vi "sub vi - Syringe Settings.vi"(7 "VISA resource name":refnum<visa-resource-name>="COM11", 9 "Flow Rate (ul/min)":dbl=100.0, 10 "Force (1-100)":dbl=100.0, 11 "Diameter (mm)":dbl=100.0) -> (0 "Accumulated Volume (ul)":dbl format="%#_6f", 1 "Flow Rate (ul/min)":dbl format="%#_6f", 2 "force setting (0-100)":dbl format="%#_6f", 3 "Diameter (mm)":dbl format="%#_6f")   [LabVIEW 2010]
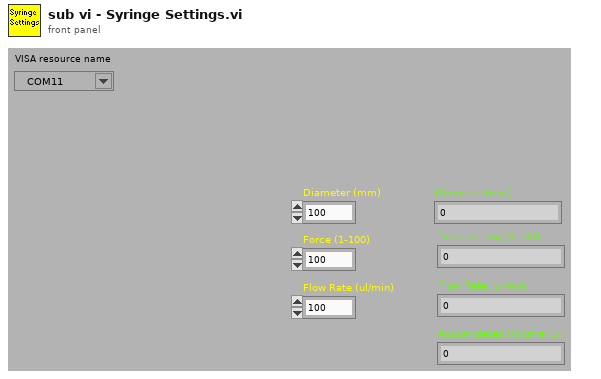
[diagram p1: front panel]
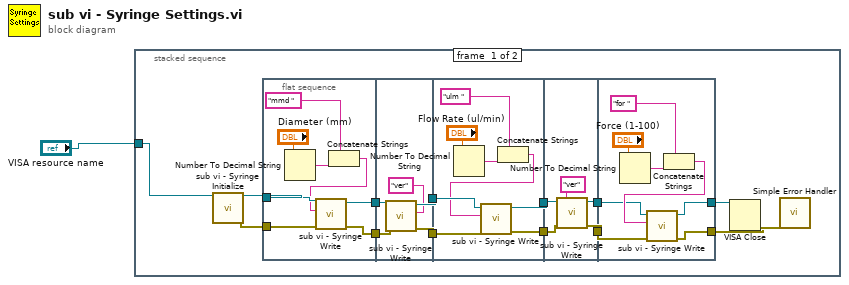
[diagram p0: block diagram]
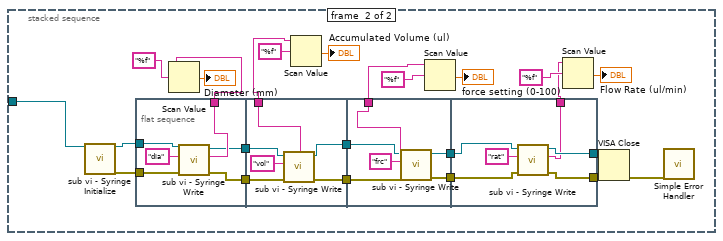
[diagram p2: hidden frame]
diagram:
  n1 = stacked-sequence {
    tunnel: "VISA resource name" -> [w2 w50]
    frame #0 {
      n2 = call "sub vi - Syringe Initialize.vi"("VISA resource name"=w2) -> ("VISA resource name out"=w6:refnum<visa-resource-name>, "error out"=w5:errorcluster)  [unwired: 13 out]
      n3 = flat-sequence {
        tunnel: w6 -> [w23]
        tunnel: w5 -> [w22]
        tunnel: [w21] -> w15
        tunnel: [w20] -> w14
        tunnel: w15 -> [w27]
        tunnel: w14 -> [w28]
        tunnel: [w26] -> w13
        tunnel: [w25] -> w12
        tunnel: w13 -> [w35]
        tunnel: w12 -> [w36]
        tunnel: [w30] -> w11
        tunnel: [w29] -> w10
        tunnel: w11 -> [w37]
        tunnel: w10 -> [w40]
        tunnel: [w38] -> w9
        tunnel: [w39] -> w8
        tunnel: [w42] -> w3
        tunnel: [w43] -> w4
        tunnel: w9 -> [w44]
        tunnel: w8 -> [w45]
        frame #0 {
          n4 = Number To Decimal String(number="Diameter (mm)") -> (decimal integer string=w17:string)  [unwired: 1 out]
          n5 = Concatenate Strings("mmd " ("string"), w17) -> (w16:string)
          n6 = call "sub vi - Syringe Write.vi"("error out"=w22, "Command"=w16, "VISA resource name out"=w23) -> ("error out 2"=w20:errorcluster, "VISA resource name out 2"=w21:refnum<visa-resource-name>)  [unwired: 7 out]
        }
        frame #1 {
          n7 = call "sub vi - Syringe Write.vi"("error out"=w28, "Command"="ver", "VISA resource name out"=w27) -> ("error out 2"=w25:errorcluster, "VISA resource name out 2"=w26:refnum<visa-resource-name>)  [unwired: 7 out]
        }
        frame #2 {
          n8 = Number To Decimal String(number="Flow Rate (ul/min)") -> (decimal integer string=w32:string)  [unwired: 1 out]
          n9 = Concatenate Strings("ulm " ("string"), w32) -> (w31:string)
          n10 = call "sub vi - Syringe Write.vi"("error out"=w36, "Command"=w31, "VISA resource name out"=w35) -> ("error out 2"=w29:errorcluster, "VISA resource name out 2"=w30:refnum<visa-resource-name>)  [unwired: 7 out]
        }
        frame #3 {
          n11 = call "sub vi - Syringe Write.vi"("error out"=w40, "Command"="ver", "VISA resource name out"=w37) -> ("error out 2"=w39:errorcluster, "VISA resource name out 2"=w38:refnum<visa-resource-name>)  [unwired: 7 out]
        }
        frame #4 {
          n12 = Number To Decimal String(number="Force (1-100)") -> (decimal integer string=w48:string)  [unwired: 1 out]
          n13 = Concatenate Strings("for " ("string"), w48) -> (w46:string)
          n14 = call "sub vi - Syringe Write.vi"("error out"=w45, "Command"=w46, "VISA resource name out"=w44) -> ("error out 2"=w42:errorcluster, "VISA resource name out 2"=w43:refnum<visa-resource-name>)  [unwired: 7 out]
        }
      }
      n15 = VISA Close(VISA resource name=w4, error in (no error)=w3) -> (error out=w7:errorcluster)
      n16 = call <vilib>:"Simple Error Handler.vi"("error in (no error)"=w7) -> ()  [unwired: 1 in, 8 out]
    }
    frame #1 {
      n17 = call "sub vi - Syringe Initialize.vi"("VISA resource name"=w50) -> ("VISA resource name out"=w55:refnum<visa-resource-name>, "error out"=w54:errorcluster)  [unwired: 13 out]
      n18 = flat-sequence {
        tunnel: [w78] -> w62
        tunnel: w55 -> [w77]
        tunnel: w54 -> [w76]
        tunnel: [w75] -> w73
        tunnel: [w74] -> w72
        tunnel: [w84] -> w57
        tunnel: w73 -> [w83]
        tunnel: w72 -> [w82]
        tunnel: [w81] -> w71
        tunnel: [w80] -> w70
        tunnel: [w88] -> w56
        tunnel: w71 -> [w87]
        tunnel: w70 -> [w86]
        tunnel: [w90] -> w69
        tunnel: [w89] -> w68
        tunnel: [w95] -> w63
        tunnel: [w96] -> w64
        tunnel: w69 -> [w93]
        tunnel: w68 -> [w94]
        tunnel: [w92] -> w51
        frame #0 {
          n19 = call "sub vi - Syringe Write.vi"("error out"=w76, "Command"="dia", "VISA resource name out"=w77) -> ("error out 2"=w74:errorcluster, "Return String"=w78:string, "VISA resource name out 2"=w75:refnum<visa-resource-name>)  [unwired: 6 out]
        }
        frame #1 {
          n20 = call "sub vi - Syringe Write.vi"("error out"=w82, "Command"="vol", "VISA resource name out"=w83) -> ("error out 2"=w81:errorcluster, "Return String"=w84:string, "VISA resource name out 2"=w80:refnum<visa-resource-name>)  [unwired: 6 out]
        }
        frame #2 {
          n21 = call "sub vi - Syringe Write.vi"("error out"=w87, "Command"="frc", "VISA resource name out"=w86) -> ("error out 2"=w89:errorcluster, "Return String"=w88:string, "VISA resource name out 2"=w90:refnum<visa-resource-name>)  [unwired: 6 out]
        }
        frame #3 {
          n22 = call "sub vi - Syringe Write.vi"("error out"=w94, "Command"="rat", "VISA resource name out"=w93) -> ("error out 2"=w95:errorcluster, "Return String"=w92:string, "VISA resource name out 2"=w96:refnum<visa-resource-name>)  [unwired: 6 out]
        }
      }
      n23 = Scan Value(string=w62, format string="%f") -> (value=→"Diameter (mm)":dbl)  [unwired: 2 out]
      n24 = Scan Value(string=w57, format string="%f") -> (value=→"Accumulated Volume (ul)":dbl)  [unwired: 2 out]
      n25 = Scan Value(string=w56, format string="%f") -> (value=→"force setting (0-100)":dbl)  [unwired: 2 out]
      n26 = Scan Value(string=w51, format string="%f") -> (value=→"Flow Rate (ul/min)":dbl)  [unwired: 2 out]
      n27 = VISA Close(VISA resource name=w64, error in (no error)=w63) -> (error out=w67:errorcluster)
      n28 = call <vilib>:"Simple Error Handler.vi"("error in (no error)"=w67) -> ()  [unwired: 1 in, 8 out]
    }
  }
